vi "Configure Ethernet.vi"(6 "default gateway":string, 7 "subnet mask":string, 8 "error in (no error)":errorcluster, 9 "ip address":string, 10 "dhcp":u16(ring) items=["disabled", "enabled"], 11 "VGC in":refnum<class "PL Inficon VGC.lvclass">) -> (0 "error out":errorcluster, 1 "ip address":string, 2 "dhcp":u16(ring) items=["disabled", "enabled"], 3 "VGC out":refnum<class "PL Inficon VGC.lvclass">, 4 "default gateway":string, 5 "subnet mask":string)   [LabVIEW 2015, in "PL Inficon VGC.lvclass"]
doc: "Configures Ethernet."
uses:
  PL Inficon VGC.lvclass
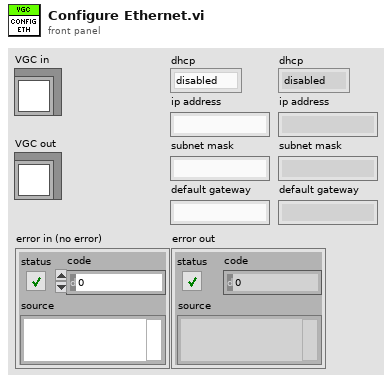
[diagram p1: front panel]
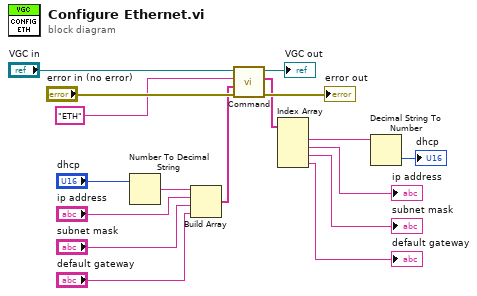
[diagram p0: block diagram]
diagram:
  n1 = Number To Decimal String(number="dhcp") -> (decimal integer string=w13:string)  [unwired: 1 in]
  n2 = Build Array(w13, "ip address", "subnet mask", "default gateway") -> (w12:string[])
  n3 = call "Command.vi"("error in (no error)"="error in (no error)", "parameters"=w12, "command"="ETH" ("format string"), "VGC in"="VGC in") -> ("error out"=→"error out":errorcluster, "response data"=w5:string[], "VGC out"=→"VGC out":refnum<class "PL Inficon VGC.lvclass">)  [unwired: 5 in]
  n4 = Index Array(array=w5) -> (element #1=w6:string, element #2=→"ip address":string, element #3=→"subnet mask":string, element #4=→"default gateway":string)  [unwired: 4 in]
  n5 = Decimal String To Number(string=w6) -> (number=→"dhcp":i32)  [unwired: 2 in, 1 out]
